vi "Flattened String to Hex.vi"(1 "Flattened String":string) -> (0 "Hex":string)   [LabVIEW 2017, in "Configit.lvlib"]
uses:
  Configit.lvlib
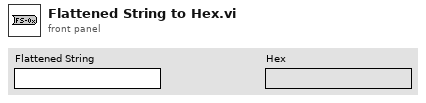
[diagram p1: front panel]
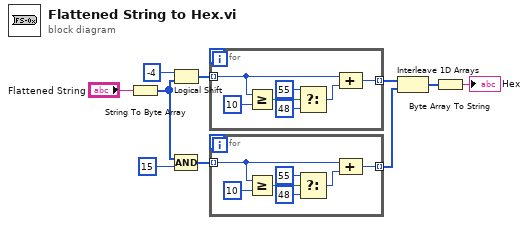
[diagram p0: block diagram]
diagram:
  n1 = String To Byte Array(string="Flattened String") -> (unsigned byte array=w8:u8[])
  n2 = Logical Shift(y=i16 -4, x=w8) -> (x << y=w4:u8[])
  n3 = Compound Arithmetic op=AND(w8, u8 15) -> (w6:u8[])
  n4 = for {
    tunnel: w4 -> [w15] mode=indexing
    tunnel: [w17] -> w1 mode=indexing
    n5 = Greater Or Equal?(x=w15, y=u8 10) -> (x >= y?=w13:bool)
    n6 = Select(t=u8 55 ("value"), s=w13, f=u8 48 ("value")) -> (s? t:f=w16:u8)
    n7 = Compound Arithmetic op=ADD(w15, w16) -> (w17:u8)
  }
  n8 = for {
    tunnel: w6 -> [w22] mode=indexing
    tunnel: [w24] -> w3 mode=indexing
    n9 = Greater Or Equal?(x=w22, y=u8 10) -> (x >= y?=w20:bool)
    n10 = Select(t=u8 55 ("value"), s=w20, f=u8 48 ("value")) -> (s? t:f=w23:u8)
    n11 = Compound Arithmetic op=ADD(w22, w23) -> (w24:u8)
  }
  n12 = Interleave 1D Arrays(w1, w3) -> (w2:u8[])
  n13 = Byte Array To String(unsigned byte array=w2) -> (string=→"Hex":string)
